vi "DivideSGL.vi"(8 "Input Valid":bool, 10 "b":sgl, 11 "a":sgl[](array[numeric])=[0.0, 0.0, 0.0, 0.0]) -> (0 "Output Valid":bool, 3 "a/b":sgl[](array[numeric]))   [LabVIEW 2014]
doc: "<b> Latency = 28 Ticks </b>"
uses:
  <vilib>/rvi/FXPMathLib/basic elements/FxpDiscreteDelay/XNode/nifxpmath_DiscreteDelay.xnode
panel:
  # "Copyright 2014 Vidrio Technologies\nScanImage 5 software is licensed under the Apache License, Version 2.0 (the \"License\"); you may not use any files contained\nwithin the ScanImage 5 release except in compliance with the License. You may obtain a copy of the License at\n http://www.apache.org/licenses/LICENSE-2.0\nUnless required by applicable law or agreed to in writing, software distributed under the License is distributed on an\n\"AS IS\" BASIS, WITHOUT WARRANTIES OR CONDITIONS OF ANY KIND, either express or implied. See the License for the\n specific language governing permissions and limitations under the License."
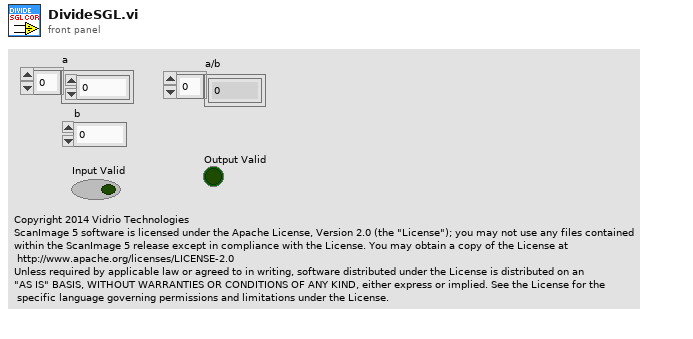
[diagram p1: front panel]
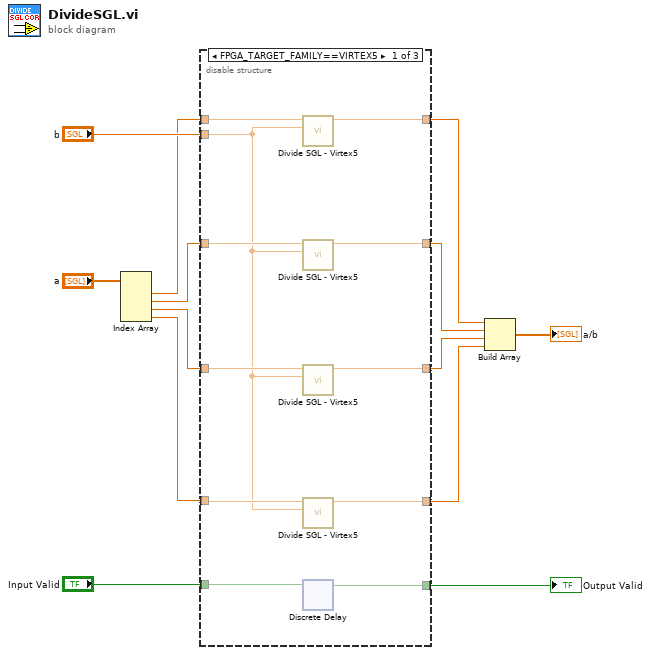
[diagram p0: block diagram]
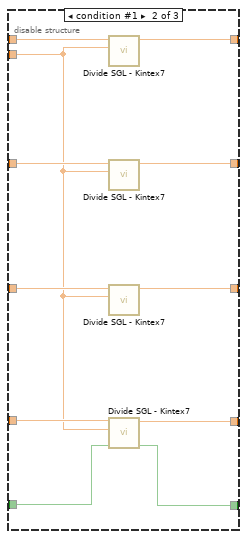
[diagram p2: hidden frame]
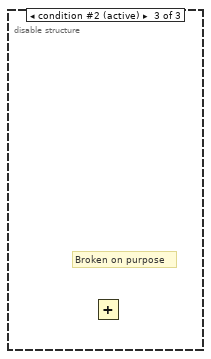
[diagram p3: hidden frame]
diagram:
  n1 = Index Array(array="a") -> (element #1=w9:sgl, element #2=w8:sgl, element #3=w6:sgl, element #4=w7:sgl)  [unwired: 4 in]
  n2 = disable-structure shown="FPGA_TARGET_FAMILY==VIRTEX5" {
    disable-tunnel: "Input Valid" -> [w24 w26 _]
    disable-tunnel: [w23 w25 _] -> w12
    disable-tunnel: "b" -> [w17 w30 _]
    disable-tunnel: w9 -> [w22 w35 _]
    disable-tunnel: w8 -> [w20 w33 _]
    disable-tunnel: w7 -> [w18 w31 _]
    disable-tunnel: w6 -> [w19 w32 _]
    disable-tunnel: [w21 w34 _] -> w5
    disable-tunnel: [w14 w29 _] -> w4
    disable-tunnel: [w15 w28 _] -> w3
    disable-tunnel: [w16 w27 _] -> w2
    frame condition #0 {
      n3 = call "Divide SGL - Virtex5.vi"("A"=w22, "B"=w17) -> ("Result"=w21:sgl)  [unwired: 7 in, 1 out]
      n4 = call "Divide SGL - Virtex5.vi"("A"=w20, "B"=w17) -> ("Result"=w14:sgl)  [unwired: 7 in, 1 out]
      n5 = call "Divide SGL - Virtex5.vi"("A"=w19, "B"=w17) -> ("Result"=w15:sgl)  [unwired: 7 in, 1 out]
      n6 = call "Divide SGL - Virtex5.vi"("A"=w18, "B"=w17) -> ("Result"=w16:sgl)  [unwired: 7 in, 1 out]
      n7 = xnode "Discrete Delay"("D"=w24) -> ("Q"=w23:bool)
    }
    frame condition #1 {
      n8 = call "Divide SGL - Kintex7.vi"("A"=w35, "B"=w30) -> ("Result"=w34:sgl)  [unwired: 7 in, 1 out]
      n9 = call "Divide SGL - Kintex7.vi"("A"=w33, "B"=w30) -> ("Result"=w29:sgl)  [unwired: 7 in, 1 out]
      n10 = call "Divide SGL - Kintex7.vi"("A"=w32, "B"=w30) -> ("Result"=w28:sgl)  [unwired: 7 in, 1 out]
      n11 = call "Divide SGL - Kintex7.vi"("A"=w31, "B"=w30, "Data Valid In"=w26) -> ("Result"=w27:sgl, "Data Valid Out"=w25:bool)  [unwired: 6 in]
    }
    frame condition #2 (active) {
      # "Broken on purpose"
      n12 = Add() -> ()  [unwired: 2 in, 1 out]
    }
  }
  "Output Valid" <- w12
  n13 = Build Array(w5, w4, w3, w2) -> (→"a/b":sgl[])
